vi "Calculator.vi"(0 "Object_and_Instance_In":T1, 5 "A":dbl, 7 "B":dbl, 9 "Calculate":bool, 11 "Error_In":errorcluster) -> (4 "Object_and_instance_Out":T1, 6 "C":dbl, 15 "Error_Out":errorcluster)   [LabVIEW 2021]
doc: "This is the core calculator Vi which performs math calculation using the calculator class."
uses:
  Controls/Queue_Operation_Select.ctl
  Drivers/QD_Main.vi
  Controls/State_and_Data.ctl
  Drivers/QD_Calci.vi
  Classes/Calculator/Calculator.lvclass
  Controls/Calculator_Data.ctl
  Controls/Object_and_instance.ctl
panel:
  out "Instance":string
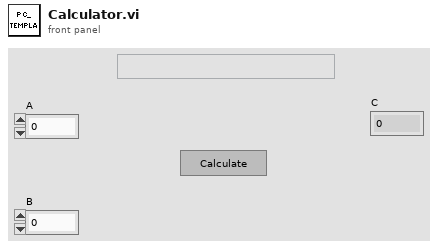
[diagram p1: front panel]
types:
  T1 = typedef "Object_and_instance.ctl" = cluster{"Object":refnum<class "Calculator.lvclass">, "Instance":string}
  T2 = typedef "Calculator_Data.ctl" = cluster{"Inputs":dbl[], "Output":dbl, "Instance":string, "Object_and_instance":T1}
  T3 = typedef "Queue_Operation_Select.ctl" = enum16{"Obtain_Queue", "Enqueue", "Enqueue_First", "Enqueue_N", "Lossy_Enqueue", "Preview", "Queue_Status", "Dequeue", "Flush", "Release_Queue"}
  T4 = typedef "State_and_Data.ctl" = cluster{"State":string, "Data":variant}
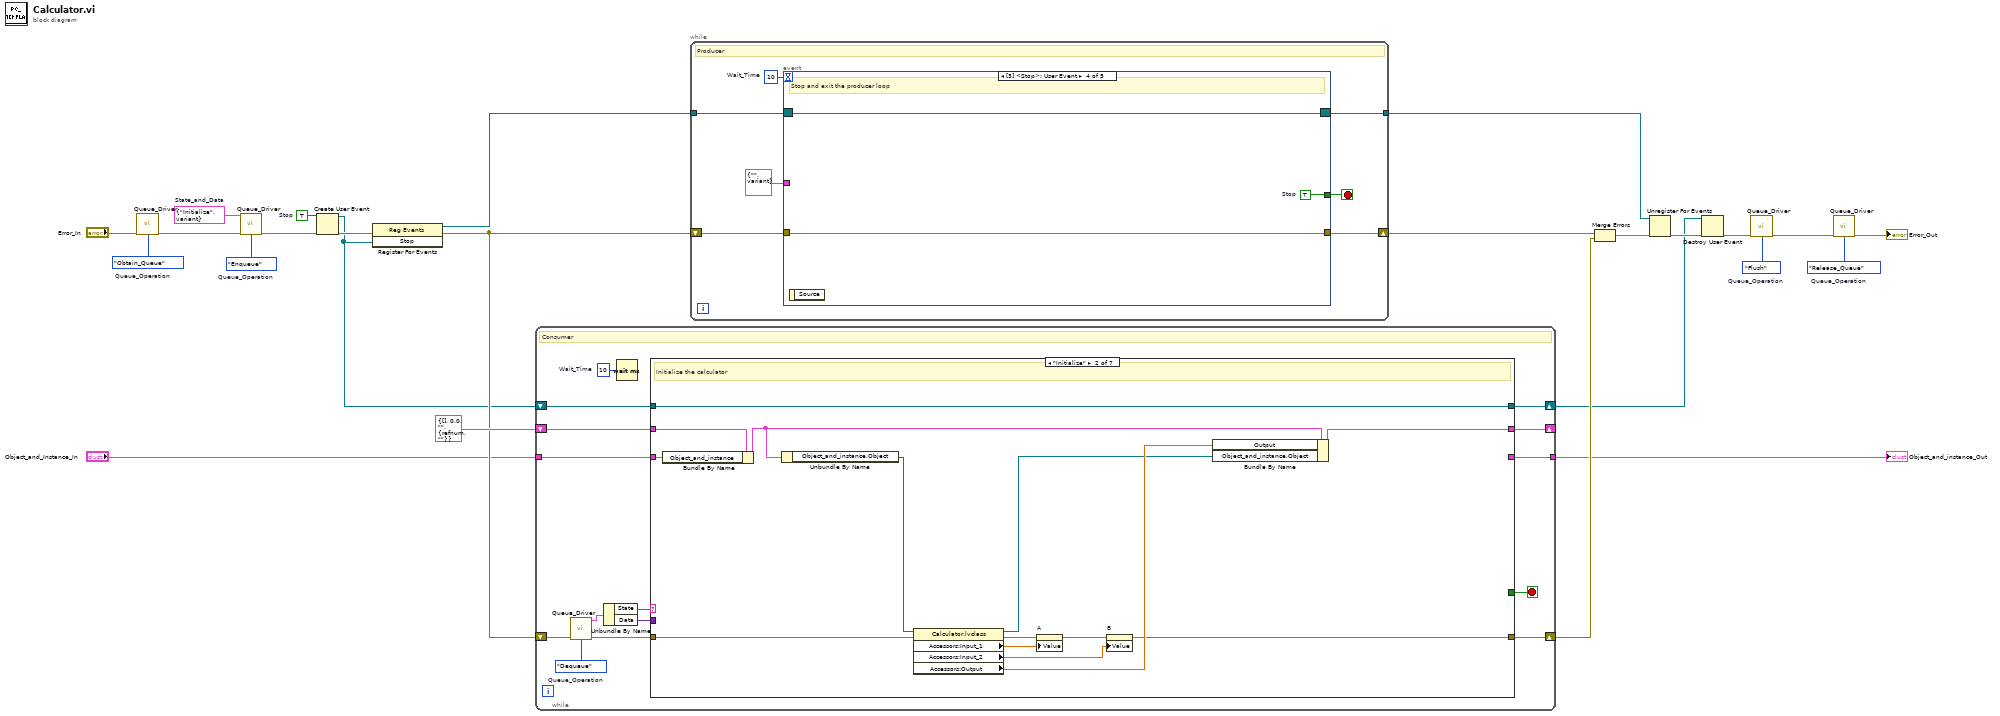
[diagram p0: block diagram]
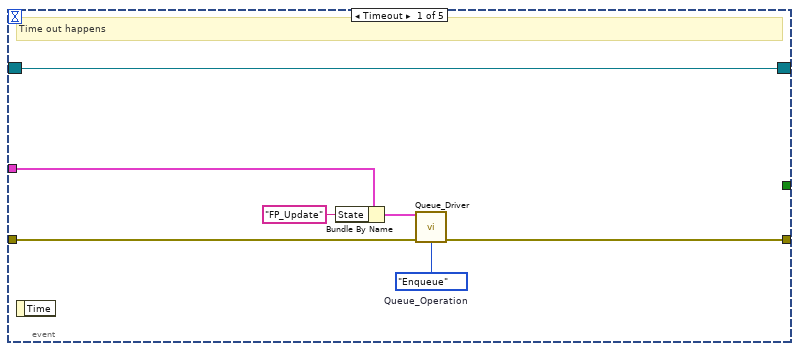
[diagram p2: hidden frame]
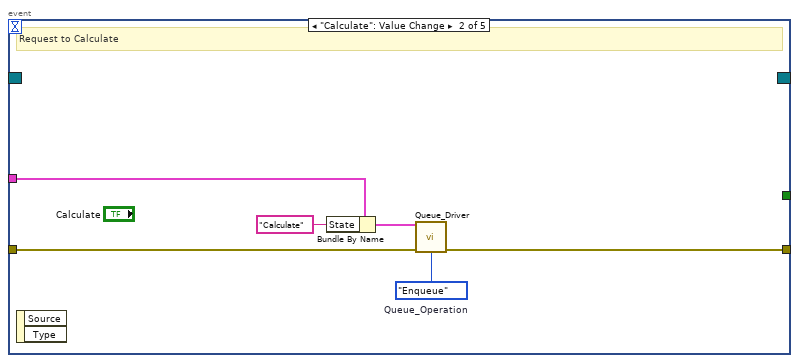
[diagram p3: hidden frame]
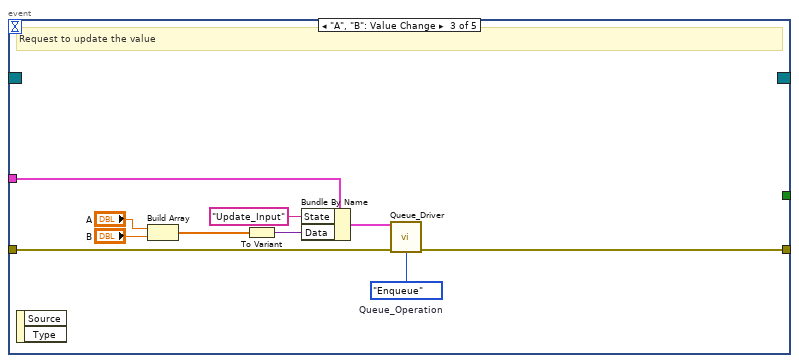
[diagram p4: hidden frame]
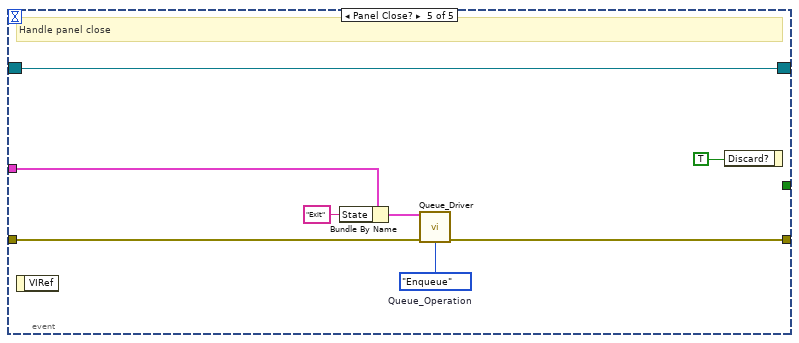
[diagram p5: hidden frame]
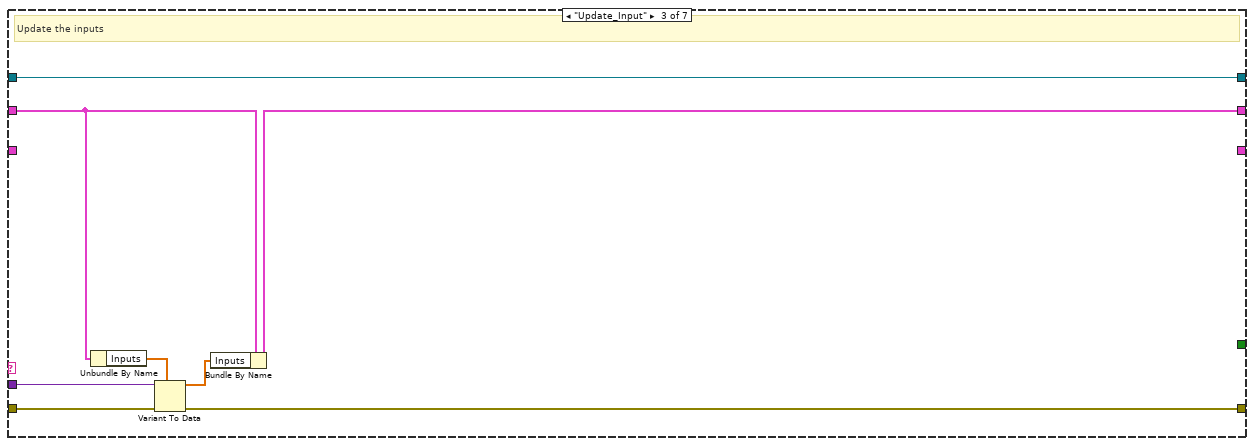
[diagram p7: hidden frame]
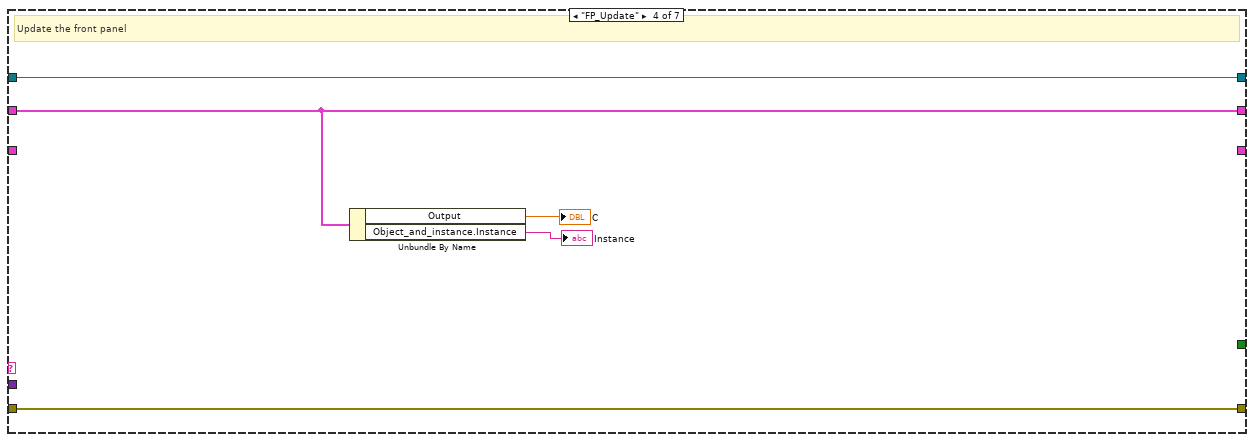
[diagram p8: hidden frame]
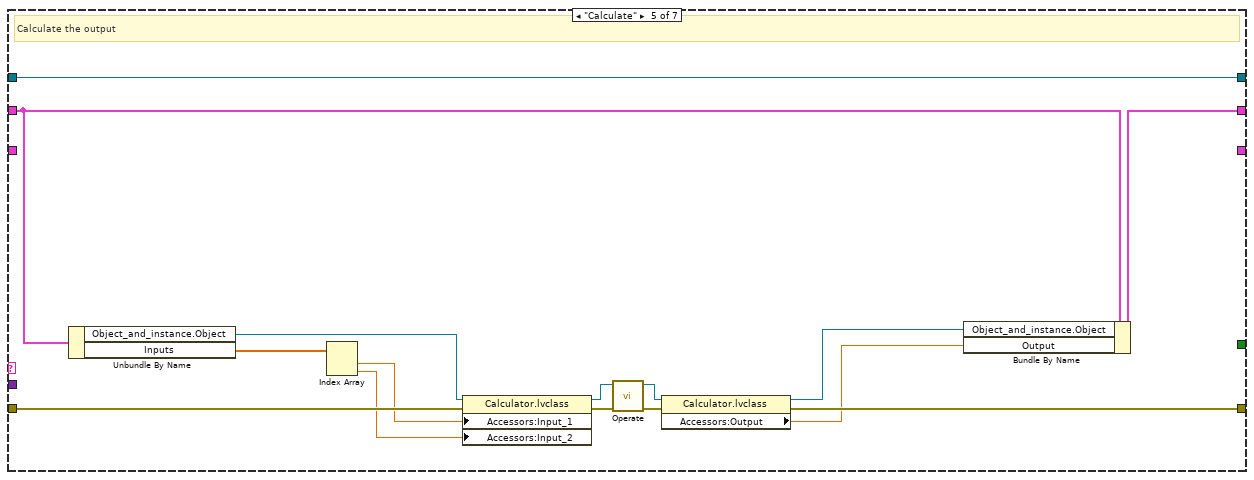
[diagram p9: hidden frame]
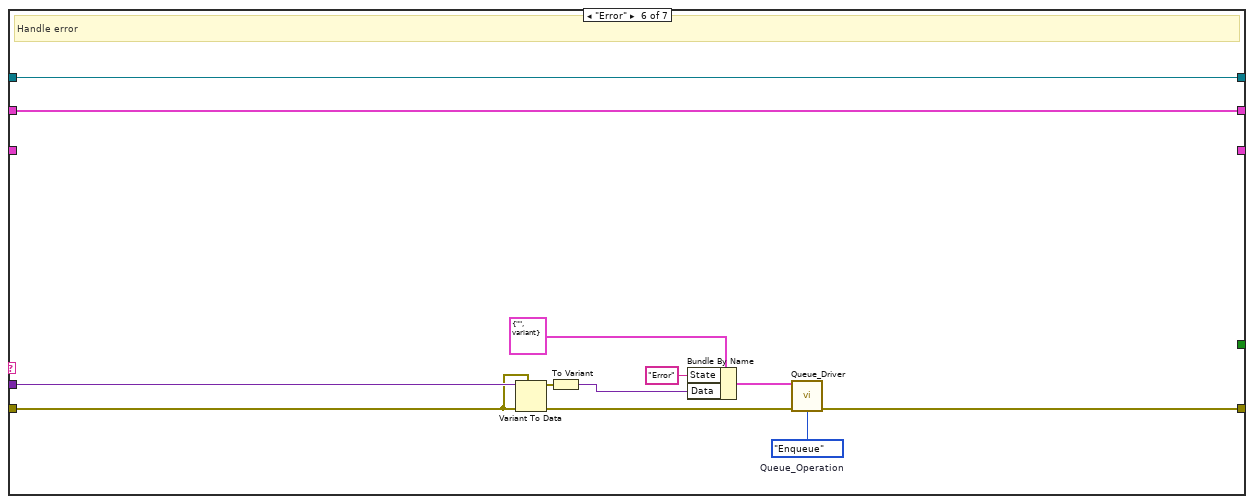
[diagram p10: hidden frame]
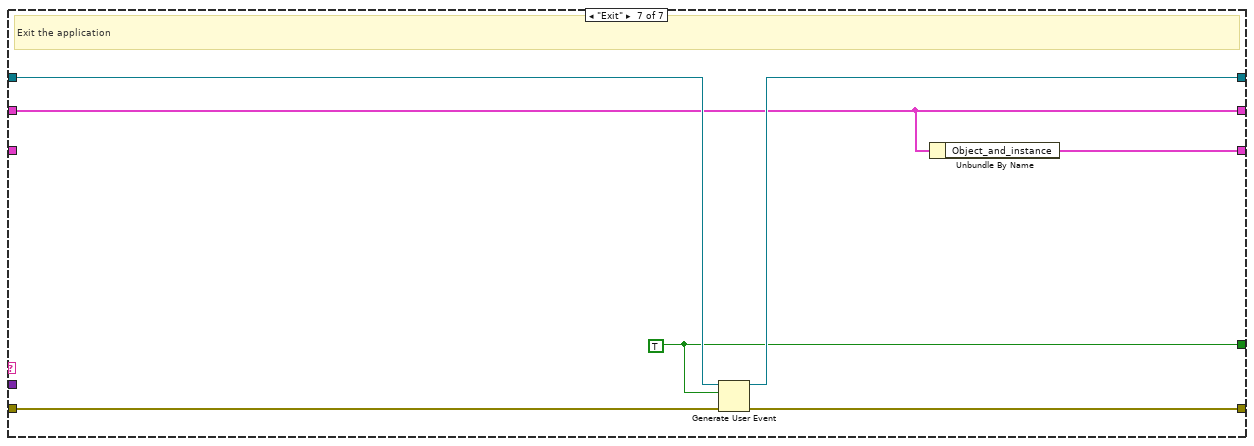
[diagram p11: hidden frame]
diagram:
  w7 = Queue_Operation_Select."Release_Queue"  # Queue_Operation
  w8 = Queue_Operation_Select."Flush"  # Queue_Operation
  w18 = TRUE  # Stop
  w21 = T4 {"State"="Initialize", "Data"=variant}  # State_and_Data
  w22 = Queue_Operation_Select."Enqueue"  # Queue_Operation
  w23 = Queue_Operation_Select."Obtain_Queue"  # Queue_Operation
  n1 = call-poly "Queue_Driver.vi"("Error_In"="Error_In", "Queue_Operation"=w23) -> ("Error_Out"=w24:errorcluster)  [unwired: 11 in, 2 out]
  n2 = call-poly "Queue_Driver.vi"("State_and_Data_In"=w21, "Error_In"=w24, "Queue_Operation"=w22) -> ("Error_Out"=w6:errorcluster)  [unwired: 10 in, 2 out]
  n3 = Create User Event(user event datatype=w18, error in=w6) -> (user event=w3:refnum<user-event>, error out=w19:errorcluster)
  n4 = register-events(error in=w19, w3) -> (reference out=w17:refnum<event-registration>, error out=w4:errorcluster)  [unwired: 1 in]
  n5 = while {
    shift-right: [w32] -> w11
    shift-left: w3 -> [w33]
    shift-right: [w31] -> _
    shift-left: T2 {"Inputs"=[], "Output"=0.0, "Instance"="", "Object_and_instance"={"Object"=refnum, "Instance"=""}} -> [w34]
    shift-right: [w30] -> w15
    shift-left: w4 -> [w40]
    tunnel: "Object_and_Instance_In" -> [w27]
    tunnel: [w26] -> w1
    stop <- w29 stop-if-true
    w28 = u32 10  # Wait_Time
    w38 = Queue_Operation_Select."Dequeue"  # Queue_Operation
    # "Consumer"
    n6 = call-poly "Queue_Driver.vi"("Error_In"=w40, "Queue_Operation"=w38) -> ("State_and_Data_Out"=w37:T4, "Error_Out"=w39:errorcluster)  [unwired: 11 in, 1 out]
    n7 = Unbundle By Name(w37) -> ("State"=w36:string, "Data"=w35:variant)
    n8 = Wait (ms)(milliseconds to wait=w28) -> ()  [unwired: 1 out]
    n9 = case shown="\"Initialize\"" w36 {
      tunnel: [w43 w45 w63 w70 w75 w93 w103] -> w30
      tunnel: w39 -> [w43 w56 w65 w70 w80 w95 w104]
      tunnel: w35 -> [_ _ w62 _ _ w96 _]
      tunnel: w34 -> [w42 w55 w61 w68 w84 w94 w99]
      tunnel: [w42 w50 w59 w68 w82 w94 w99] -> w31
      tunnel: w33 -> [w41 w57 w64 w69 w85 w97 w102]
      tunnel: [w41 w57 w64 w69 w85 w97 w101] -> w32
      tunnel: [_ _ _ _ _ _ w100] -> w29
      tunnel: w27 -> [_ w48 _ _ _ _ _]
      tunnel: [_ _ _ _ _ _ w98] -> w26
      frame Default {
      }
      frame "Initialize" {
        # "Initialize the calculator"
        n10 = Bundle By Name(cluster=w55, "Object_and_instance"=w48) -> (w47:T2)
        n11 = Unbundle By Name(w47) -> ("Object_and_instance.Object"=w46:refnum<class "Calculator.lvclass">)
        n12 = property class="Calculator.lvclass"(reference=w46, error in=w56) -> (reference out=w44:refnum<class "Calculator.lvclass">, error out=w54:errorcluster, "Accessors:Input_1"=w52:dbl, "Accessors:Input_2"=w51:dbl, "Accessors:Output"=w49:dbl)
        n13 = property on="A" class="DigNum (strict)"(error in=w54, "Value"=w52) -> (error out=w53:errorcluster)  [unwired: 1 in, 1 out]
        n14 = property on="B" class="DigNum (strict)"(error in=w53, "Value"=w51) -> (error out=w45:errorcluster)  [unwired: 1 in, 1 out]
        n15 = Bundle By Name(cluster=w47, "Output"=w49, "Object_and_instance.Object"=w44) -> (w50:T2)
      }
      frame "Update_Input" {
        # "Update the inputs"
        n16 = Unbundle By Name(w61) -> ("Inputs"=w60:dbl[])
        n17 = Variant To Data(error in=w65, type=w60, Variant=w62) -> (data=w58:dbl[], error out=w63:errorcluster)
        n18 = Bundle By Name(cluster=w61, "Inputs"=w58) -> (w59:T2)
      }
      frame "FP_Update" {
        # "Update the front panel"
        n19 = Unbundle By Name(w68) -> ("Output"=→"C":dbl, "Object_and_instance.Instance"=→"Instance":string)
      }
      frame "Calculate" {
        # "Calculate the output"
        n20 = Unbundle By Name(w84) -> ("Object_and_instance.Object"=w72:refnum<class "Calculator.lvclass">, "Inputs"=w83:dbl[])
        n21 = Index Array(array=w83) -> (element #1=w77:dbl, element #2=w76:dbl)  [unwired: 2 in]
        n22 = property class="Calculator.lvclass"(reference=w72, error in=w80, "Accessors:Input_1"=w77, "Accessors:Input_2"=w76) -> (reference out=w78:refnum<class "Calculator.lvclass">, error out=w79:errorcluster)
        n23 = call-dynamic "Operate.vi"("Error_In"=w79, "Calculator_In"=w78) -> ("Error_Out"=w81:errorcluster, "Calculator_Out"=w74:refnum<class "Calculator.lvclass">)  [unwired: 8 in]
        n24 = property class="Calculator.lvclass"(reference=w74, error in=w81) -> (reference out=w71:refnum<class "Calculator.lvclass">, error out=w75:errorcluster, "Accessors:Output"=w73:dbl)
        n25 = Bundle By Name(cluster=w84, "Object_and_instance.Object"=w71, "Output"=w73) -> (w82:T2)
      }
      frame "Error" {
        w92 = Queue_Operation_Select."Enqueue"  # Queue_Operation
        # "Handle error"
        n26 = Variant To Data(error in=w95, type=w95, Variant=w96) -> (data=w87:errorcluster, error out=w91:errorcluster)
        n27 = To Variant(anything=w87) -> (Variant=w86:variant)
        n28 = Bundle By Name(cluster=T4 {"State"="", "Data"=variant} ("State_and_Data"), "State"="Error", "Data"=w86) -> (w89:T4)
        n29 = call-poly "Queue_Driver.vi"("State_and_Data_In"=w89, "Error_In"=w91, "Queue_Operation"=w92) -> ("Error_Out"=w93:errorcluster)  [unwired: 10 in, 2 out]
      }
      frame "Exit" {
        w100 = TRUE
        # "Exit the application"
        n30 = Generate User Event(user event=w102, event data cluster=w100, error in=w104) -> (user event out=w101:refnum<user-event>, error out=w103:errorcluster)  [unwired: 1 in]
        n31 = Unbundle By Name(w99) -> ("Object_and_instance"=w98:T1)
      }
    }
  }
  "Object_and_instance_Out" <- w1
  n32 = while {
    tunnel: w17 -> [w110]
    shift-right: [w109] -> w16
    shift-left: w4 -> [w111]
    tunnel: [w107] -> w13
    stop <- w106 stop-if-true
    w108 = 10  # Wait_Time
    # "Producer"
    n33 = event shown="[3] <Stop>: User Event" {
      selector: w110 -> [w118 _ _ w135 w139]
      dyn-events: [w118 _ _ w135 w139] -> w107
      timeout: w108 -> [_ _ _ _ _]
      tunnel: w111 -> [w114 w121 w131 w136 w142]
      tunnel: [w113 w120 w130 w136 w141] -> w109
      tunnel: [_ _ _ w137 _] -> w106
      tunnel: T4 {"State"="", "Data"=variant} ("State_and_Data") -> [w112 w119 w125 _ w138]
      event Timeout {
        w116 = Queue_Operation_Select."Enqueue"  # Queue_Operation
        # "Time out happens"
        n34 = event-data() -> ()  [unwired: 1 in, 1 out]
        n35 = Bundle By Name(cluster=w112, "State"="FP_Update") -> (w115:T4)
        n36 = call-poly "Queue_Driver.vi"("State_and_Data_In"=w115, "Error_In"=w114, "Queue_Operation"=w116) -> ("Error_Out"=w113:errorcluster)  [unwired: 10 in, 2 out]
      }
      event "Calculate": Value Change {
        w123 = Queue_Operation_Select."Enqueue"  # Queue_Operation
        # "Request to Calculate"
        n37 = event-data() -> ()  [unwired: 1 in, 2 out]
        n38 = Bundle By Name(cluster=w119, "State"="Calculate") -> (w122:T4)
        n39 = call-poly "Queue_Driver.vi"("State_and_Data_In"=w122, "Error_In"=w121, "Queue_Operation"=w123) -> ("Error_Out"=w120:errorcluster)  [unwired: 10 in, 2 out]
      }
      event "A", "B": Value Change {
        w133 = Queue_Operation_Select."Enqueue"  # Queue_Operation
        # "Request to update the value"
        n40 = event-data() -> ()  [unwired: 1 in, 2 out]
        n41 = Build Array("A", "B") -> (w127:dbl[])
        n42 = To Variant(anything=w127) -> (Variant=w126:variant)
        n43 = Bundle By Name(cluster=w125, "State"="Update_Input", "Data"=w126) -> (w132:T4)
        n44 = call-poly "Queue_Driver.vi"("State_and_Data_In"=w132, "Error_In"=w131, "Queue_Operation"=w133) -> ("Error_Out"=w130:errorcluster)  [unwired: 10 in, 2 out]
      }
      event User Event {
        w137 = TRUE  # Stop
        # "Stop and exit the producer loop"
        n45 = event-data() -> ()  [unwired: 1 in, 1 out]
      }
      event Panel Close? {
        w143 = Queue_Operation_Select."Enqueue"  # Queue_Operation
        # "Handle panel close"
        n46 = event-data() -> ()  [unwired: 1 in, 1 out]
        n47 = Bundle By Name(cluster=w138, "State"="Exit") -> (w140:T4)
        n48 = call-poly "Queue_Driver.vi"("State_and_Data_In"=w140, "Error_In"=w142, "Queue_Operation"=w143) -> ("Error_Out"=w141:errorcluster)  [unwired: 10 in, 2 out]
        n49 = event-data("Discard?"=TRUE) -> ()  [unwired: 1 in, 1 out]
      }
    }
  }
  n50 = Merge Errors(w16, w15) -> (w14:errorcluster)
  n51 = Unregister For Events(event registration refnum=w13, error in=w14) -> (error out=w12:errorcluster)
  n52 = Destroy User Event(user event=w11, error in=w12) -> (error out=w10:errorcluster)
  n53 = call-poly "Queue_Driver.vi"("Error_In"=w10, "Queue_Operation"=w8) -> ("Error_Out"=w9:errorcluster)  [unwired: 11 in, 2 out]
  n54 = call-poly "Queue_Driver.vi"("Error_In"=w9, "Queue_Operation"=w7) -> ("Error_Out"=→"Error_Out":errorcluster)  [unwired: 11 in, 2 out]
